vi "ReadTableHead.vi"(11 "theadString":string) -> (3 "theadData":string[](array[string]))   [LabVIEW 2013]
uses:
  <vilib>/regexp/Match Regular Expression.xnode
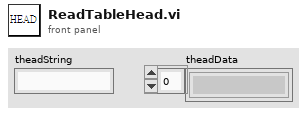
[diagram p1: front panel]
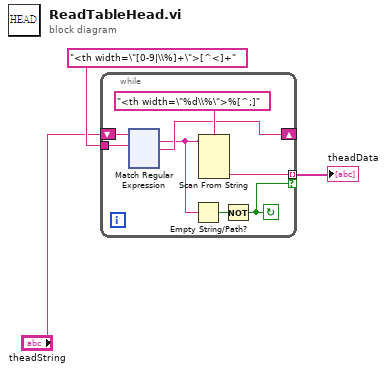
[diagram p0: block diagram]
diagram:
  n1 = while {
    tunnel: "<th width=\"[0-9|\\%]+\">[^<]+" ("regular expression") -> [w10]
    shift-right: [w7] -> _
    shift-left: "theadString" -> [w11]
    tunnel: [w8] -> w3 mode=indexing if=w4
    stop <- w4 continue-if-true
    n2 = xnode "Match Regular Expression"("input string"=w11, "regular expression"=w10) -> ("whole match"=w6:string, "after match"=w7:string)  [unwired: 4 in, 3 out]
    n3 = Empty String/Path?(string/path=w6) -> (empty?=w5:bool)
    n4 = Scan From String(format string="<th width=\"%d\\%\">%[^;]", input string=w6) -> (output 2=w8:string)  [unwired: 5 in, 3 out]
    n5 = Not(x=w5) -> (.not. x?=w4:bool)
  }
  "theadData" <- w3
